vi "half adder.vi"() -> ()   [LabVIEW 2015]
panel:
  out "carry":bool
  out "sum":bool
  in  "Boolean 2":bool
  in  "Boolean":bool
  # "half adder"
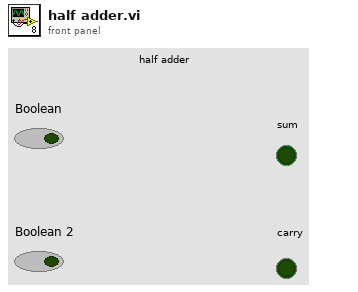
[diagram p1: front panel]
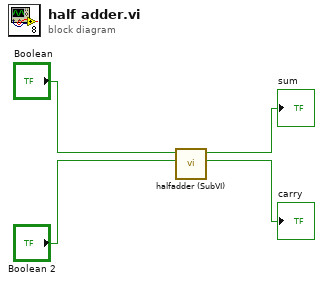
[diagram p0: block diagram]
diagram:
  n1 = call "halfadder (SubVI).vi"("Boolean 2"="Boolean 2", "Boolean"="Boolean") -> ("carry"=→"carry":bool, "sum"=→"sum":bool)  [unwired: 8 in]
